vi "Actor Core.vi"(8 "error in":errorcluster, 11 "GObject View in":refnum<class "RTM View.lvclass">) -> (0 "error out":errorcluster, 3 "Actor out":refnum<class "Actor.lvclass">)   [LabVIEW 2013, in "SET Project Editor.lvlib" / "RTM View.lvclass"]
doc: "(<B>Filename</B>: Actor Framework.lvlib:Actor.lvclass:Actor Core.vi)\n\nReceives messages to the actor, reacts to them, and initiates any error handling that may shut the actor down.\n\nDescendant classes may override this VI to append parallel tasks for the actor to complete while it handles messages. Overrides use the Call Parent Method node."
uses:
  RTM View.lvclass
  <vilib>/ActorFramework/Actor/Actor.lvclass
  <vilib>/Utility/miscctls.llb/LVRowAndColumnTypeDef.ctl
  <vilib>/ActorFramework/Actor/Actor.lvclass/Actor.ctl
  <vilib>/ActorFramework/Message Enqueuer/Message Enqueuer.lvclass/Message Enqueuer.ctl
  UI View/UI View.lvclass/UI View.ctl
  MCListbox View Messages/MCLB Request Edit Cell Msg/MCLB Request Edit Cell Msg.lvclass/MCLB Request Edit Cell Msg.ctl
  Controller Messages/Assign Shared Resource Msg/Assign Shared Resource Msg.lvclass/Assign Shared Resource Msg.ctl
  Controller Messages/Remove Object Msg/Remove Object Msg.lvclass/Remove Object Msg.ctl
  MCListbox View/MCListbox View.lvclass/MCListbox View.ctl
  RTM View.lvclass/RTM View.ctl
  MCListbox View/MCListbox View.lvclass
  MCListbox View/Properties/Write Editable From.vi
  UI View/Read UUID.vi
  <vilib>/ActorFramework/Message Enqueuer/Init from Existing Queue.vi
  <vilib>/ActorFramework/Message Enqueuer/Enqueue.vi
  <vilib>/ActorFramework/Message Priority Queue/Priority Enqueue.vi
  <vilib>/ActorFramework/Message Enqueuer/Message Enqueuer.lvclass
  <vilib>/ActorFramework/Stop Msg/Stop Msg.lvclass
  MCListbox View Messages/MCLB Request Edit Cell Msg/MCLB Request Edit Cell Msg.lvclass
  UI View Messages/Preview Msg/Preview Msg.lvclass
  Controller Messages/Assign Shared Resource Msg/Assign Shared Resource Msg.lvclass
  Controller Messages/Remove Object Msg/Remove Object Msg.lvclass
  MCListbox View Messages/MCLB StrEdit Resize Msg/MCLB StrEdit Resize Msg.lvclass
  Lib/Unicode/SET_Unicode Tools.lvlib
panel:
  in  "Preview":bool
  out "Path":string
  in  "StrEdit":string
  in  "Items":i32(listbox)
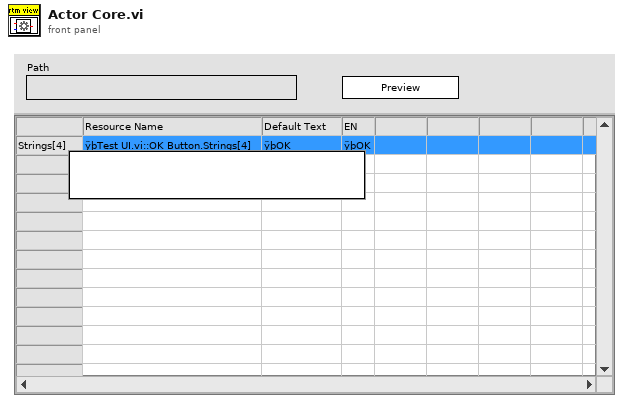
[diagram p1: front panel]
types:
  T1 = typedef "LVRowAndColumnTypeDef.ctl" = cluster{"Row":i32, "Column":i32}
  T2 = typedef "LVPoint32TypeDef.ctl" = cluster{"Horizontal":i32, "Vertical":i32}
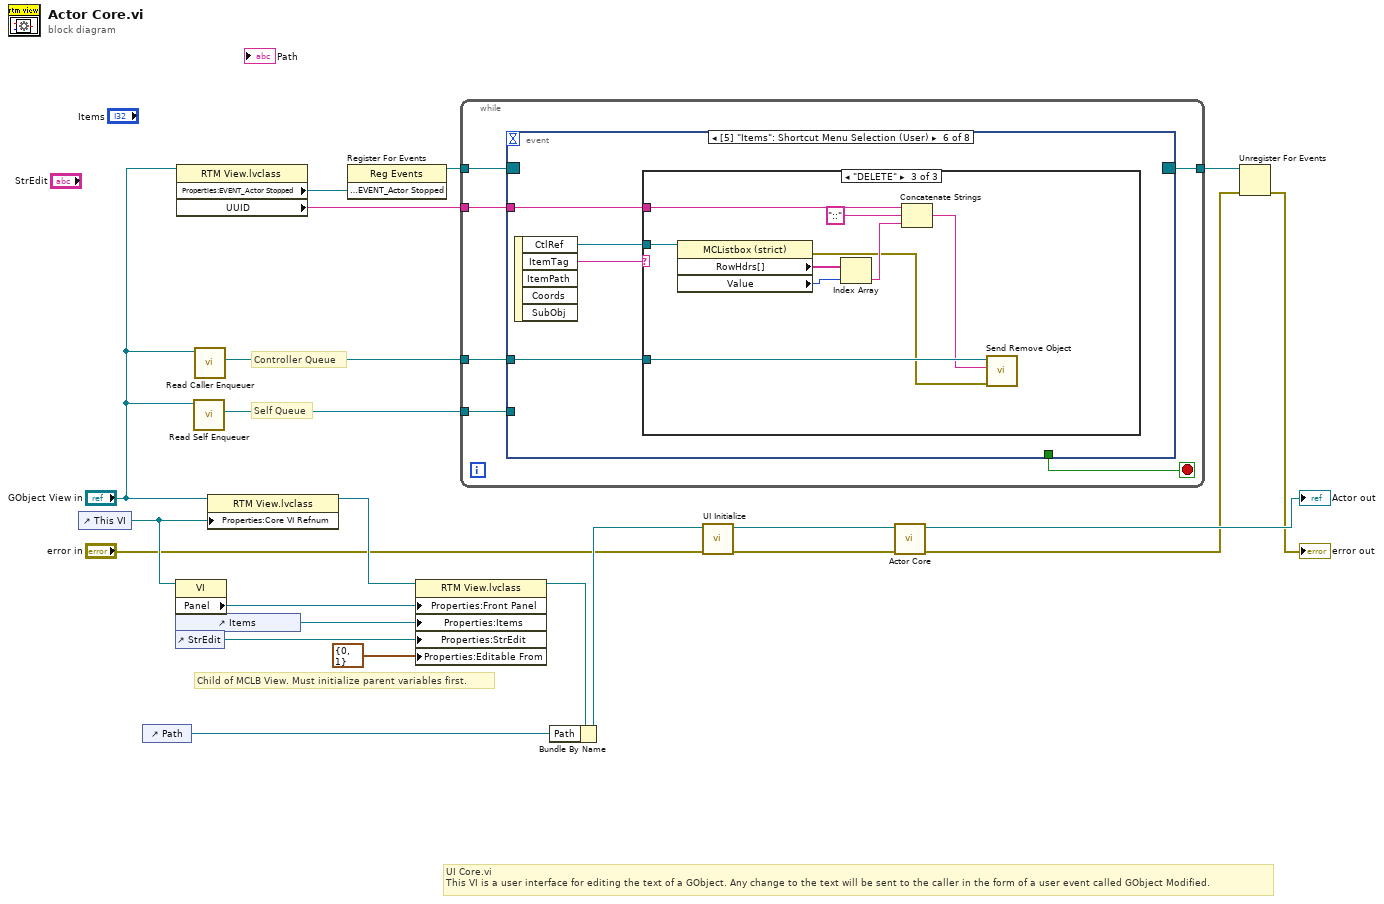
[diagram p0: block diagram]
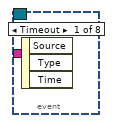
[diagram p2: hidden frame]
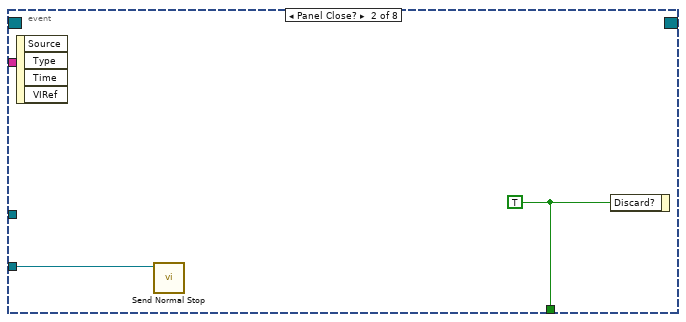
[diagram p3: hidden frame]
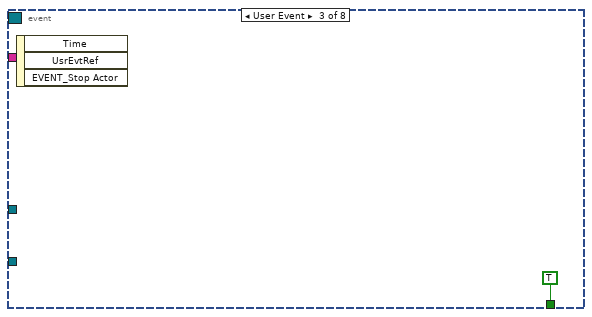
[diagram p4: hidden frame]
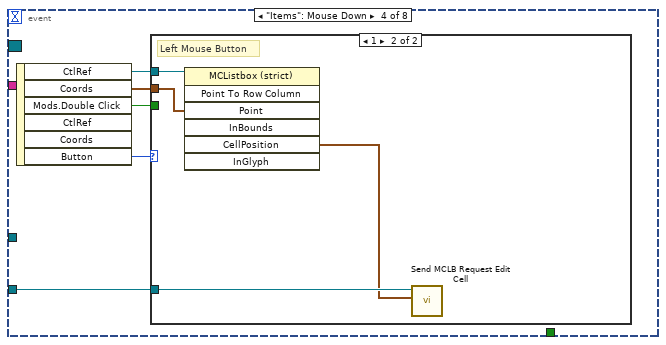
[diagram p5: hidden frame]
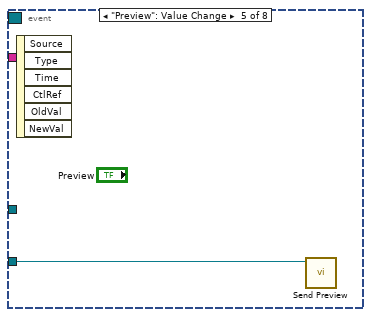
[diagram p7: hidden frame]
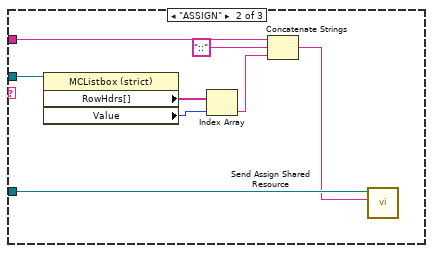
[diagram p9: hidden frame]
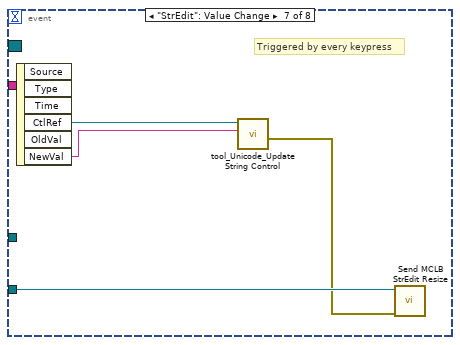
[diagram p10: hidden frame]
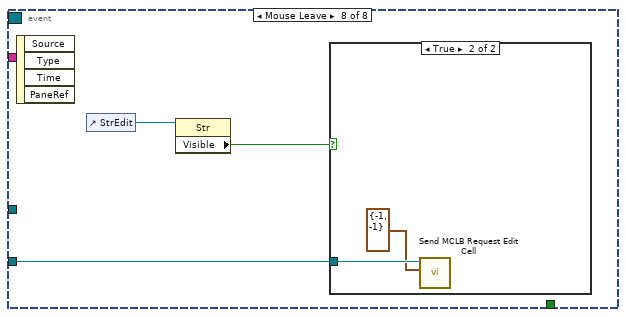
[diagram p11: hidden frame]
diagram:
  # "Child of MCLB View. Must initialize parent variables first."
  # "Controller Queue"
  # "UI Core.vi\nThis VI is a user interface for editing the text of a GObject. Any change to the text will be sent to the caller in the form of a user event called GObject Modified."
  # "Self Queue"
  n1 = control-ref of="This VI"() -> (w14:refnum<vi>)
  n2 = control-ref of="Path"() -> (w13:refnum<vi>)
  n3 = property class="VI"(reference=w14) -> ("Panel"=w10:refnum<vi>)  [unwired: 1 in, 2 out]
  n4 = control-ref of="Items"() -> (w9:refnum<vi>)
  n5 = control-ref of="StrEdit"() -> (w8:refnum<vi>)
  n6 = property class="RTM View.lvclass"(reference="GObject View in") -> ("Properties:EVENT_Actor Stopped"=w21:refnum<user-event>, "UUID"=w1:string)  [unwired: 1 in, 2 out]
  n7 = call <vilib>:"Read Self Enqueuer.vi"("Actor"="GObject View in") -> ("Self Enqueuer"=w12:refnum<class "Message Enqueuer.lvclass">)  [unwired: 10 in]
  n8 = call <vilib>:"Read Caller Enqueuer.vi"("Actor"="GObject View in") -> ("Caller Enqueuer"=w16:refnum<class "Message Enqueuer.lvclass">)  [unwired: 10 in]
  n9 = property class="RTM View.lvclass"(reference="GObject View in", "Properties:Core VI Refnum"=w14) -> (reference out=w11:refnum<class "RTM View.lvclass">)  [unwired: 1 in, 1 out]
  n10 = register-events(w21) -> (reference out=w20:refnum<event-registration>)  [unwired: 2 in, 1 out]
  n11 = property class="RTM View.lvclass"(reference=w11, "Properties:Front Panel"=w10, "Properties:Items"=w9, "Properties:StrEdit"=w8, "Properties:Editable From"=T1 {"Row"=0, "Column"=1} ("Editable From")) -> (reference out=w7:refnum<class "RTM View.lvclass">)  [unwired: 1 in, 1 out]
  n12 = while {
    tunnel: w20 -> [w27]
    tunnel: [w26] -> w19
    tunnel: w12 -> [w25]
    tunnel: w16 -> [w24]
    tunnel: w1 -> [w23]
    stop <- w28 stop-if-true
    n13 = event shown="[5] \"Items\": Shortcut Menu Selection (User)" {
      selector: w27 -> [_ _ _ _ _ _ _ _]
      dyn-events: [_ _ _ _ _ _ _ _] -> w26
      timeout: _ -> [_ _ _ _ _ _ _ _]
      tunnel: [_ w30 TRUE ("Discard?") _ _ _ _ _] -> w28
      tunnel: w25 -> [_ w29 _ w32 w41 _ w64 w67]
      tunnel: w24 -> [_ _ _ _ _ w44 _ _]
      tunnel: w23 -> [_ _ _ _ _ w42 _ _]
      event Timeout {
        n14 = event-data() -> ()  [unwired: 1 in, 3 out]
      }
      event Panel Close? {
        w30 = TRUE ("Discard?")
        n15 = event-data() -> ()  [unwired: 1 in, 4 out]
        n16 = call <vilib>:"Send Normal Stop.vi"("Message Enqueuer"=w29) -> ()  [unwired: 10 in, 1 out]
        n17 = event-data("Discard?"=w30) -> ()  [unwired: 1 in, 1 out]
      }
      event User Event {
        n18 = event-data() -> ()  [unwired: 1 in, 3 out]
      }
      event "Items": Mouse Down {
        n19 = event-data() -> ("CtlRef"=w35:refnum<vi>, "Coords"=w34:T2, "Mods.Double Click"=w33:bool, "Button"=w36:u16)  [unwired: 1 in, 2 out]
        n20 = case shown="1" w36 {
          tunnel: w35 -> [_ w40]
          tunnel: w34 -> [_ w39]
          tunnel: w33 -> [_ _]
          tunnel: w32 -> [_ w38]
          frame 0, Default {
          }
          frame 1 {
            # "Left Mouse Button"
            n21 = invoke class="MCListbox (strict)" method="Point To Row Column"(reference=w40, "Point"=w39) -> ("CellPosition"=w37:T1)  [unwired: 5 in, 6 out]
            n22 = call "Send MCLB Request Edit Cell.vi"("RowAndCollumn"=w37, "Message Enqueuer"=w38) -> ()  [unwired: 8 in, 2 out]
          }
        }
      }
      event "Preview": Value Change {
        n23 = event-data() -> ()  [unwired: 1 in, 6 out]
        n24 = call "Send Preview.vi"("Message Enqueuer"=w41) -> ()  [unwired: 9 in, 2 out]
      }
      event "Items": Shortcut Menu Selection (User) {
        n25 = event-data() -> ("CtlRef"=w43:refnum<vi>, "ItemTag"=w45:string)  [unwired: 1 in, 3 out]
        n26 = case shown="\"DELETE\"" w45 {
          tunnel: w44 -> [_ w53 w56]
          tunnel: w43 -> [_ w52 w62]
          tunnel: w42 -> [_ w49 w59]
          frame Default {
          }
          frame "ASSIGN" {
            n27 = property class="MCListbox (strict)"(reference=w52) -> ("RowHdrs[]"=w51:string[], "Value"=w50:i32)  [unwired: 1 in, 2 out]
            n28 = Index Array(array=w51, index=w50) -> (element=w47:string)
            n29 = Concatenate Strings(w49, "::" ("string"), w47) -> (w46:string)
            n30 = call "Send Assign Shared Resource.vi"("UID"=w46, "Message Enqueuer"=w53) -> ()  [unwired: 8 in, 2 out]
          }
          frame "DELETE" {
            n31 = property class="MCListbox (strict)"(reference=w62) -> (error out=w54:errorcluster, "RowHdrs[]"=w61:string[], "Value"=w60:i32)  [unwired: 1 in, 1 out]
            n32 = Index Array(array=w61, index=w60) -> (element=w57:string)
            n33 = Concatenate Strings(w59, "::" ("string"), w57) -> (w55:string)
            n34 = call "Send Remove Object.vi"("error in (no error)"=w54, "UUID"=w55, "Message Enqueuer"=w56) -> ()  [unwired: 7 in, 2 out]
          }
        }
      }
      event "StrEdit": Value Change {
        # "Triggered by every keypress"
        n35 = event-data() -> ("CtlRef"=w66:refnum<vi>, "NewVal"=w65:string)  [unwired: 1 in, 4 out]
        n36 = call "tool_Unicode_Update String Control.vi"("String (UTF-16)"=w65, "*StrControl in"=w66) -> ("error out"=w63:errorcluster)  [unwired: 8 in, 1 out]
        n37 = call "Send MCLB StrEdit Resize.vi"("error in (no error)"=w63, "Message Enqueuer"=w64) -> ()  [unwired: 8 in, 2 out]
      }
      event Mouse Leave {
        n38 = event-data() -> ()  [unwired: 1 in, 4 out]
        n39 = control-ref of="StrEdit"() -> (w69:refnum<vi>)
        n40 = property class="Str"(reference=w69) -> ("Visible"=w68:bool)  [unwired: 1 in, 2 out]
        n41 = case shown="True" w68 {
          tunnel: w67 -> [_ w71]
          frame False {
          }
          frame True {
            n42 = call "Send MCLB Request Edit Cell.vi"("RowAndCollumn"=T1 {"Row"=-1, "Column"=-1} ("Cell Position"), "Message Enqueuer"=w71) -> ()  [unwired: 8 in, 2 out]
          }
        }
      }
    }
  }
  n43 = Bundle By Name(cluster=w7, "Path"=w13) -> (w4:refnum<class "RTM View.lvclass">)
  n44 = call-dynamic "UI Initialize.vi"("error in (no error)"="error in", "GObject View in"=w4) -> ("error out"=w2:errorcluster, "GObject View out"=w5:refnum<class "RTM View.lvclass">)  [unwired: 8 in]
  n45 = call-parent "Actor Core.vi"("error in"=w2, "Actor in"=w5) -> ("error out"=w18:errorcluster, "Actor out"=→"Actor out":refnum<class "Actor.lvclass">)  [unwired: 8 in]
  n46 = Unregister For Events(event registration refnum=w19, error in=w18) -> (error out=→"error out":errorcluster)
